vi "Execute Command.vi"(8 "error in (no error)":errorcluster, 10 "UI Command Manager Stop in":refnum<class "UI Command Manager Stop.lvclass">, 11 "User Interface References":T1={"This VI"=refnum, "User Interace Plugin"=refnum, "UI Picture Container References"={"Header Image"=refnum, "Footer Image"=refnum}, "Sliding Menu XControl"=refnum, "Menu Container"=refnum, "UI Configuration Information"={"Space Between Buttons"=3, "Number of Buttons to Show"=6, "Header Image"=path "Images/Blue Background.bmp", "Footer Image"=path "Images/Blue Background.bmp"}, "Header Text"=refnum}) -> (0 "error out":errorcluster, 1 "Stop?":bool, 2 "UI Command Manager Stop out":refnum<class "UI Command Manager Stop.lvclass">, 3 "User Interface References Out":T1={"This VI"=refnum, "User Interace Plugin"=refnum, "UI Picture Container References"={"Header Image"=refnum, "Footer Image"=refnum}, "Sliding Menu XControl"=refnum, "Menu Container"=refnum, "UI Configuration Information"={"Space Between Buttons"=3, "Number of Buttons to Show"=6, "Header Image"=path "Images/Blue Background.bmp", "Footer Image"=path "Images/Blue Background.bmp"}, "Header Text"=refnum})   [LabVIEW 2011, in "UI Command Manager Stop.lvclass"]
uses:
  UI Command Manager Stop.lvclass
  Main Type Definitions/User Interface Type Definitions.ctl
  Main Type Definitions/UI Picture Containers.ctl
  Sliding Menu/Sliding Menu Library/Sliding Menu xControl/Sliding Menu XControl.xctl
  UI Control Definitions/UI Configuration Information.ctl
  UI Command Manager.lvclass
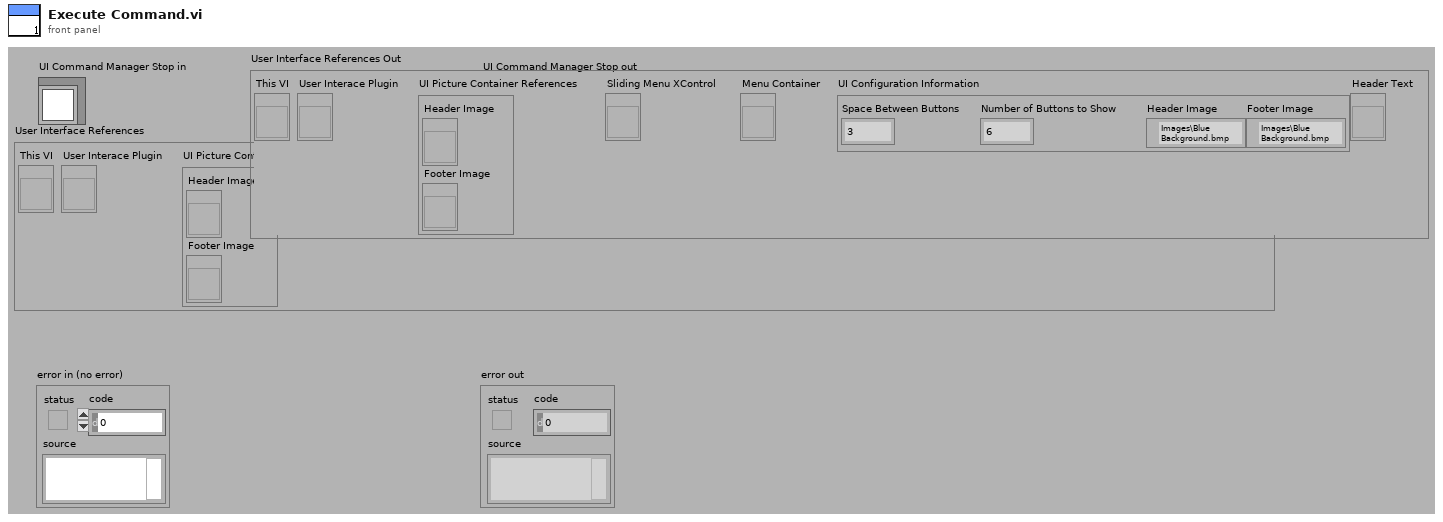
[diagram p1: front panel]
types:
  T1 = typedef "User Interface Type Definitions.ctl" = cluster{"This VI":refnum<vi>, "User Interace Plugin":refnum<vi>, "UI Picture Container References":T2, "Sliding Menu XControl":refnum<vi>, "Menu Container":refnum<vi>, "UI Configuration Information":T3, "Header Text":refnum<vi>}
  T2 = typedef "UI Picture Containers.ctl" = cluster{"Header Image":refnum<vi>, "Footer Image":refnum<vi>}
  T3 = typedef "UI Configuration Information.ctl" = cluster{"Space Between Buttons":i32, "Number of Buttons to Show":i32, "Header Image":path, "Footer Image":path}
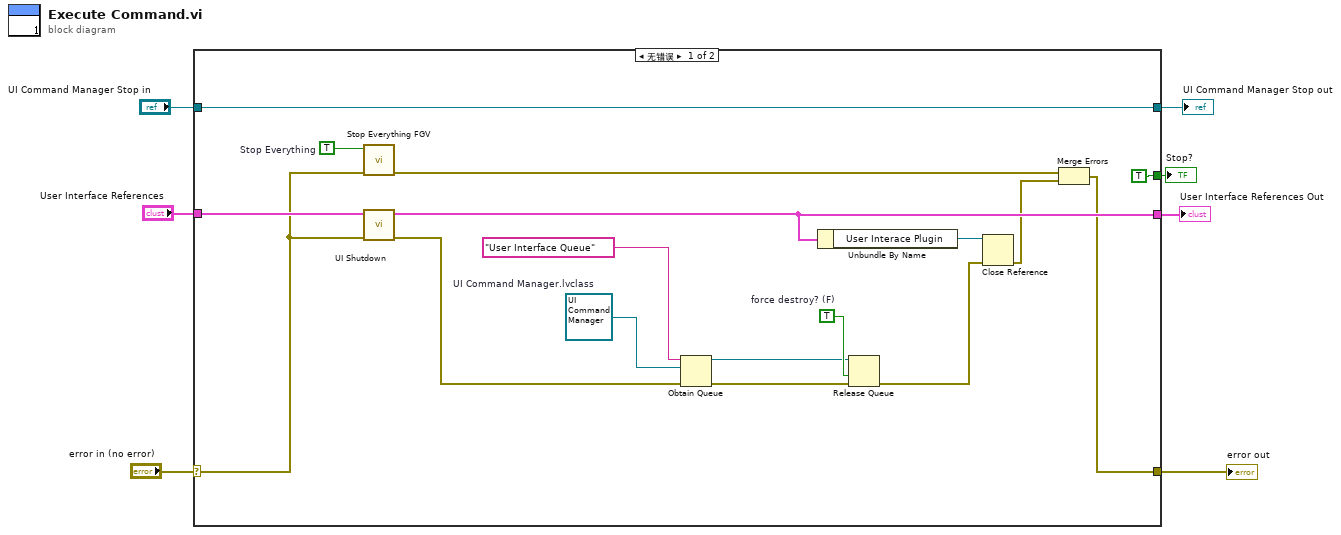
[diagram p0: block diagram]
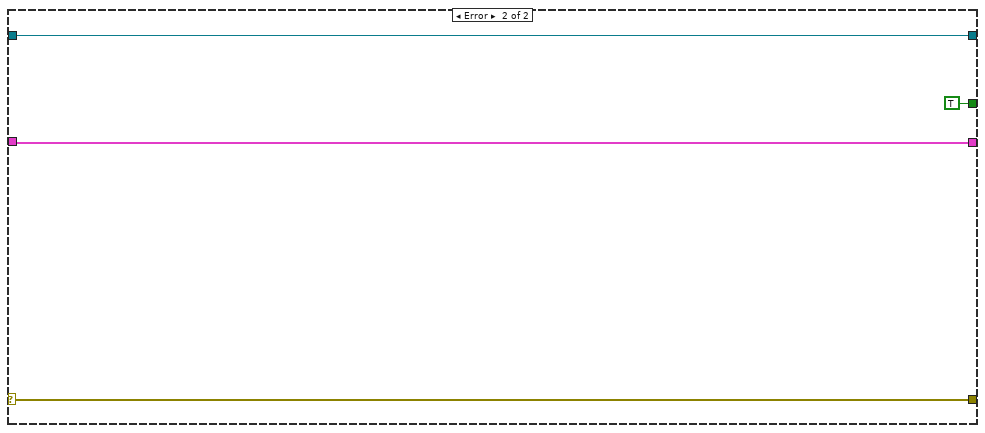
[diagram p2: hidden frame]
diagram:
  n1 = case shown="无错误" "error in (no error)" {
    selector: "error in (no error)" -> [w11 w28]
    tunnel: "User Interface References" -> [w24 w26]
    tunnel: [TRUE ("Stop?") TRUE ("Stop?")] -> w6
    tunnel: [w22 w26] -> w5
    tunnel: [w10 w28] -> w3
    tunnel: "UI Command Manager Stop in" -> [w13 w27]
    tunnel: [w13 w27] -> w1
    frame No Error {
      w12 = TRUE  # Stop Everything
      w18 = refnum<class "UI Command Manager.lvclass"> refnum  # UI Command Manager.lvclass
      w20 = TRUE  # force destroy? (F)
      n2 = call "Stop Everything FGV.vi"("error in (no error)"=w11, "Stop Everything?"=w12) -> ("error out"=w8:errorcluster)  [unwired: 8 in, 1 out]
      n3 = call "UI Shutdown.vi"("error in (no error)"=w11, "User Interface References"=w24) -> ("error out"=w15:errorcluster, "User Interface References Out"=w22:T1)  [unwired: 8 in]
      n4 = Obtain Queue(name (unnamed)="User Interface Queue", element data type=w18, error in (no error)=w15) -> (queue out=w17:refnum<queue>, error out=w16:errorcluster)  [unwired: 2 in, 1 out]
      n5 = Unbundle By Name(w22) -> ("User Interace Plugin"=w21:refnum<vi>)
      n6 = Release Queue(queue=w17, force destroy? (F)=w20, error in (no error)=w16) -> (error out=w14:errorcluster)  [unwired: 2 out]
      n7 = Close Reference(reference=w21, error in (no error)=w14) -> (error out=w9:errorcluster)
      n8 = Merge Errors(w8, w9) -> (w10:errorcluster)
    }
    frame Error {
    }
  }
  "UI Command Manager Stop out" <- w1
  "Stop?" <- w6
  "User Interface References Out" <- w5
  "error out" <- w3
